vi "Peregrine_move.vi"(0 "Handle in":refnum<visa-resource-name>, 2 "Address":u8, 5 "Target":i32, 7 "Speed":i16, 9 "Acceleration":u16, 11 "error":errorcluster) -> (4 "Handle out":refnum<visa-resource-name>, 15 "error out":errorcluster)   [LabVIEW 2019]
panel:
  out "Acceleration response":u16
  out "Speed response":i16
  out "Target response":i32
  out "Command response":i32
  out "Address response":u8
  # "Inputs"
  # "Response message\nNOT FINISHED"
  # "Output"
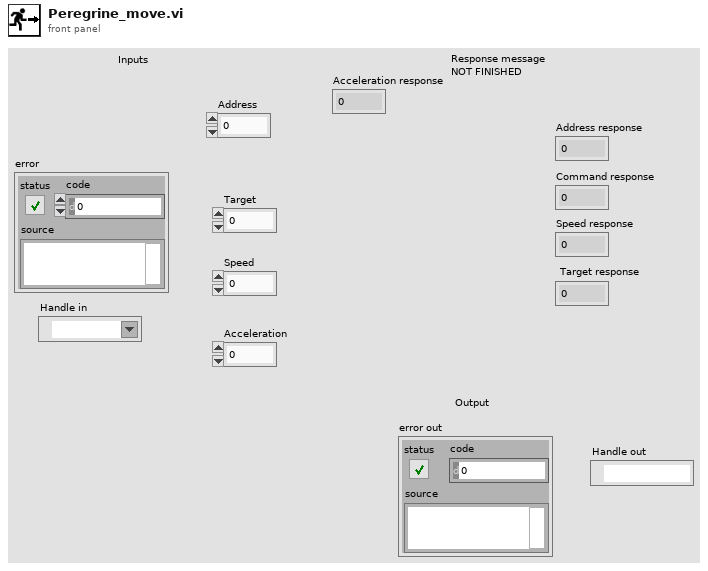
[diagram p1: front panel]
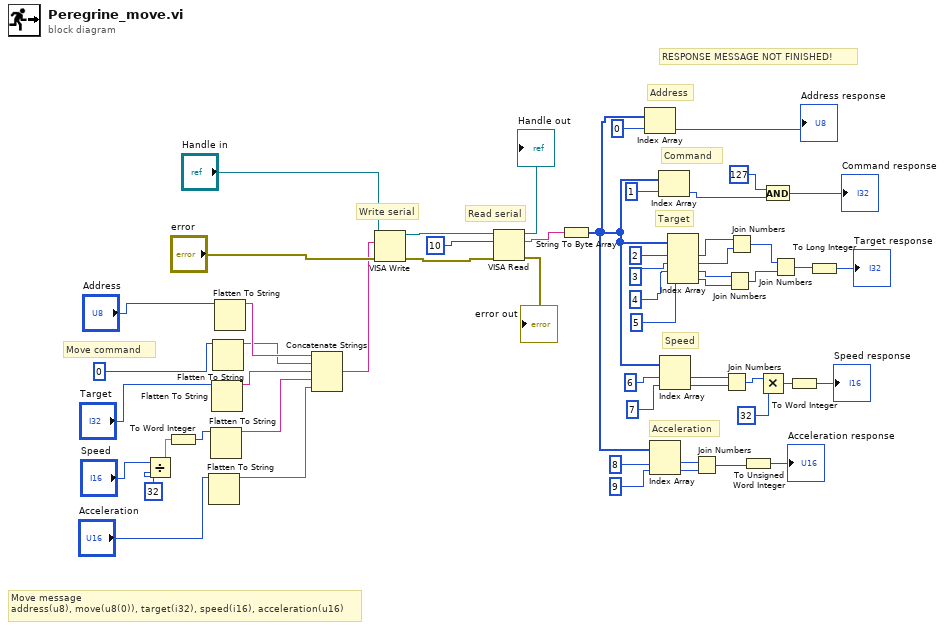
[diagram p0: block diagram]
diagram:
  # "RESPONSE MESSAGE NOT FINISHED!"
  # "Move command"
  # "Command"
  # "Address"
  # "Acceleration"
  # "Speed"
  # "Target"
  # "Read serial"
  # "Write serial"
  # "Move message\naddress(u8), move(u8(0)), target(i32), speed(i16), acceleration(u16)"
  n1 = Divide(x="Speed", y=32) -> (x/y=w7:dbl)
  n2 = To Word Integer(number=w7) -> (16bit integer=w6:i16)
  n3 = Flatten To String(anything="Acceleration") -> (data string=w11:string)  [unwired: 3 in, 2 out]
  n4 = Flatten To String(anything=w6) -> (data string=w12:string)  [unwired: 3 in, 2 out]
  n5 = Flatten To String(anything="Target") -> (data string=w13:string)  [unwired: 3 in, 2 out]
  n6 = Flatten To String(anything=u8 0) -> (data string=w14:string)  [unwired: 3 in, 2 out]
  n7 = Flatten To String(anything="Address") -> (data string=w18:string)  [unwired: 3 in, 2 out]
  n8 = Concatenate Strings(w18, w14, w13, w12, w11) -> (w10:string)
  n9 = VISA Write(VISA resource name="Handle in", write buffer=w10, error in (no error)="error") -> (VISA resource name out=w55:refnum<visa-resource-name>, error out=w20:errorcluster)  [unwired: 1 out]
  n10 = VISA Read(VISA resource name=w55, byte count=10, error in (no error)=w20) -> (VISA resource name out=→"Handle out":refnum<visa-resource-name>, read buffer=w53:string, error out=→"error out":errorcluster)  [unwired: 1 out]
  n11 = String To Byte Array(string=w53) -> (unsigned byte array=w45:u8[])
  n12 = Index Array(array=w45, index=0) -> (element=→"Address response":u8)
  n13 = Index Array(array=w45, index #1=8, index #2=9) -> (element #1=w35:u8, element #2=w34:u8)
  n14 = Index Array(array=w45, index=1) -> (element=w37:u8)
  n15 = Index Array(array=w45, index #1=6, index #2=7) -> (element #1=w30:u8, element #2=w29:u8)
  n16 = Index Array(array=w45, index #1=2, index #2=3, index #3=4, index #4=5) -> (element #1=w43:u8, element #2=w42:u8, element #3=w41:u8, element #4=w40:u8)
  n17 = Join Numbers(hi=w35, lo=w34) -> ((hi.lo)=w5:u16)
  n18 = Join Numbers(hi=w30, lo=w29) -> ((hi.lo)=w1:u16)
  n19 = Join Numbers(hi=w41, lo=w40) -> ((hi.lo)=w39:u16)
  n20 = Join Numbers(hi=w43, lo=w42) -> ((hi.lo)=w38:u16)
  n21 = To Unsigned Word Integer(number=w5) -> (unsigned 16bit integer=→"Acceleration response":u16)
  n22 = Multiply(x=w1, y=32) -> (x*y=w3:i32)
  n23 = And(x=127, y=w37) -> (x .and. y?=→"Command response":i32)
  n24 = Join Numbers(hi=w38, lo=w39) -> ((hi.lo)=w33:u32)
  n25 = To Word Integer(number=w3) -> (16bit integer=→"Speed response":i16)
  n26 = To Long Integer(number=w33) -> (32bit integer=→"Target response":i32)
